vi "ex_1_FeedbackNode.vi"() -> ()   [LabVIEW 2020]
panel:
  out "Waveform Chart":dbl(graph)
  in  "dx":dbl
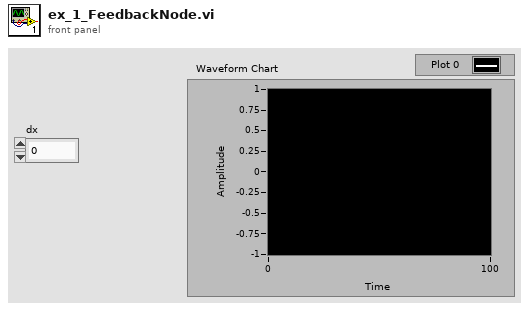
[diagram p1: front panel]
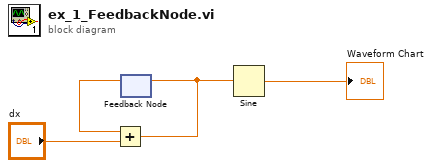
[diagram p0: block diagram]
diagram:
  n1 = feedback #1() -> (w3:dbl)  [unwired: 1 in]
  n2 = Add(x=w3, y="dx") -> (x+y=w2:dbl)
  n3 = feedback-in #1(w2) -> ()
  n4 = Sine(x=w2) -> (sin(x)=→"Waveform Chart":dbl)
